vi "Get Time.vi"() -> (2 "date/time string":string, 5 "Time Stamp":timestamp)   [LabVIEW 2015]
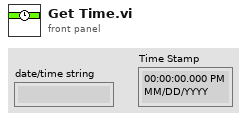
[diagram p1: front panel]
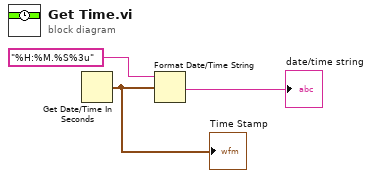
[diagram p0: block diagram]
diagram:
  n1 = Get Date/Time In Seconds() -> (seconds since 1Jan1904=w1:timestamp)
  "Time Stamp" <- w1
  n2 = Format Date/Time String(time format string (%c)="%H:%M.%S%3u", seconds (now)=w1) -> (date/time string=→"date/time string":string)  [unwired: 1 in]
